vi "Selection Color Write.vi"(4 "error in (no error)":errorcluster, 5 "Value":u32(colorbox), 6 "Container State":T3, 7 "Display State In":T1={"Persistent"={"Elements"=[], "PicElements"=[], "Limits"=[], "Selection"=[], "Selection Color"=0, "Highlight"=[], "Highlight Val"=0, "Highlight Color"={"Back"=0, "Edge"=0}, "Font"={"Details"={"Font Name:"="Lucida Sans", "Size"=24, "Strikeout?"=FALSE, "Italic?"=FALSE, "Underline?"=FALSE, "Outline?"=FALSE, "Shadow?"=FALSE, "Bold?"=TRUE}, "Color"=7697781}, "Bakground Color"=0}, "List Ref"=refnum, "nbVisible"=0, "FirstIdx"=0, "More.Width"=0}) -> (0 "error out":errorcluster, 3 "Display State Out":T1={"Persistent"={"Elements"=[], "PicElements"=[], "Limits"=[], "Selection"=[], "Selection Color"=0, "Highlight"=[], "Highlight Val"=0, "Highlight Color"={"Back"=0, "Edge"=0}, "Font"={"Details"={"Font Name:"="Lucida Sans", "Size"=24, "Strikeout?"=FALSE, "Italic?"=FALSE, "Underline?"=FALSE, "Outline?"=FALSE, "Shadow?"=FALSE, "Bold?"=TRUE}, "Color"=7697781}, "Bakground Color"=0}, "List Ref"=refnum, "nbVisible"=0, "FirstIdx"=0, "More.Width"=0})   [LabVIEW 2016, in "Horizontal MenuList.xctl"]
uses:
  Horizontal MenuList.xctl
  <vilib>/_xctls/Container State.ctl
  Horizontal MenuList_State.ctl
  _SubVIs/Highlight Colors.ctl
  <vilib>/_xctls/XControlSupport.lvlib
panel:
  # "Replace the Value Control below with a Control of desired type.\nDo not remove this Control or the others from the connector pane.\nDo not change the connector pane pattern.\nThe Value control should always be the third terminal from top on the input side in the connector pane."
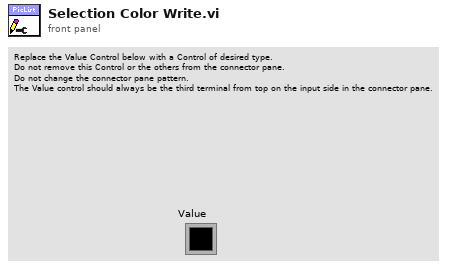
[diagram p1: front panel]
types:
  T1 = typedef "Horizontal MenuList.xctl/Horizontal MenuList_State.ctl" = cluster{"Persistent":cluster{"Elements":string[], "PicElements":picture[], "Limits":i32[], "Selection":picture[], "Selection Color":u32, "Highlight":picture[], "Highlight Val":i32, "Highlight Color":T2, "Font":cluster{"Details":cluster{"Font Name:":string, "Size":i16, "Strikeout?":bool, "Italic?":bool, "Underline?":bool, "Outline?":bool, "Shadow?":bool, "Bold?":bool}, "Color":u32}, "Bakground Color":u32}, "List Ref":refnum<vi>, "nbVisible":u8, "FirstIdx":u8, "More.Width":u8}
  T2 = typedef "Horizontal MenuList.xctl/Highlight Colors.ctl" = cluster{"Back":u32, "Edge":u32}
  T3 = typedef "XControlSupport.lvlib/Container State.ctl" = cluster{"Indicator?":bool, "Run Mode?":bool, " Refnum":refnum<vi>}
  T4 = typedef "LVBoundsTypeDef.ctl" = cluster{"Width":u32, "Height":u32}
  T5 = cluster{"left":i16, "top":i16, "right":i16, "bottom":i16}
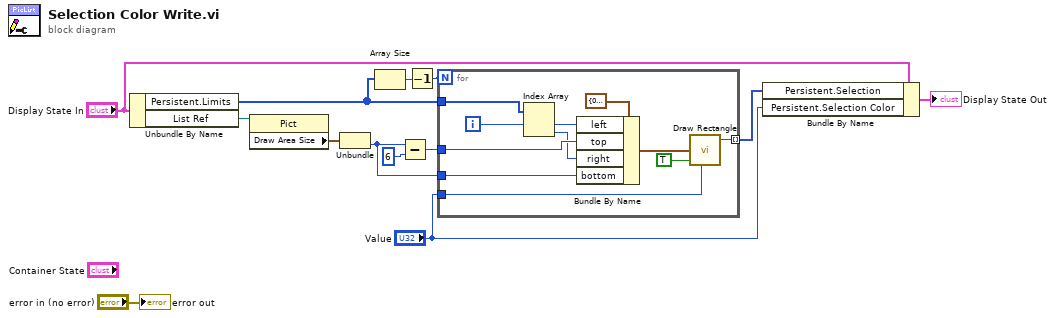
[diagram p0: block diagram]
diagram:
  n1 = Unbundle By Name("Display State In") -> ("Persistent.Limits"=w3:i32[], "List Ref"=w9:refnum<vi>)
  n2 = property class="Pict"(reference=w9) -> ("Draw Area Size"=w8:T4)  [unwired: 1 in, 2 out]
  n3 = Unbundle(w8) -> ("Height"=w6:u32)  [unwired: 1 out]
  n4 = Array Size(array=w3) -> (size(s)=w2:i32)
  n5 = Subtract(x=w6, y=u32 6) -> (x-y=w5:u32)
  n6 = Decrement(x=w2) -> (x-1=w1:i32)
  n7 = for {
    N: w1 -> [_]
    tunnel: "Value" -> [w23]
    tunnel: w6 -> [w21]
    tunnel: w5 -> [w20]
    tunnel: w3 -> [w18]
    tunnel: [w16] -> w4 mode=indexing
    i -> [w15]
    n8 = Index Array(array=w18, index #1=w15) -> (element #1=w17:i32, element #2=w14:i32)  [unwired: 1 in]
    n9 = Bundle By Name(cluster=T5 {"left"=0, "top"=0, "right"=0, "bottom"=0} ("rect"), "left"=w17, "top"=w20, "right"=w14, "bottom"=w21) -> (w19:T5)
    n10 = call <vilib>:"Draw Rectangle.vi"("rect"=w19, "fill?(F)"=TRUE, "color(black)"=w23) -> ("new picture"=w16:picture)  [unwired: 6 in]
  }
  n11 = Bundle By Name(cluster="Display State In", "Persistent.Selection"=w4, "Persistent.Selection Color"="Value") -> (→"Display State Out":T1)
  "error out" <- "error in (no error)"
